vi "List Things.vi"(8 "error in (no error)":errorcluster, 11 "IoT Session in":refnum<class "IoT Session.lvclass">) -> (0 "error out":errorcluster, 2 "Things":string[](array[string]), 3 "IoT Session out":refnum<class "IoT Session.lvclass">)   [LabVIEW 2015, in "NI_AWS_IoT.lvlib" / "IoT Session.lvclass"]
uses:
  IoT Session.lvclass
  Core/HTTP Request/Request Options.ctl
  Core/HTTP Request/Name Value Pair.ctl
  Core/HTTP Request/Region handling.ctl
  Core/HTTP Request/URL formatting.ctl
  Core/HTTP Request/HTTP Request.lvclass
  JSON Parsing/NI_JSON Parsing.lvlib
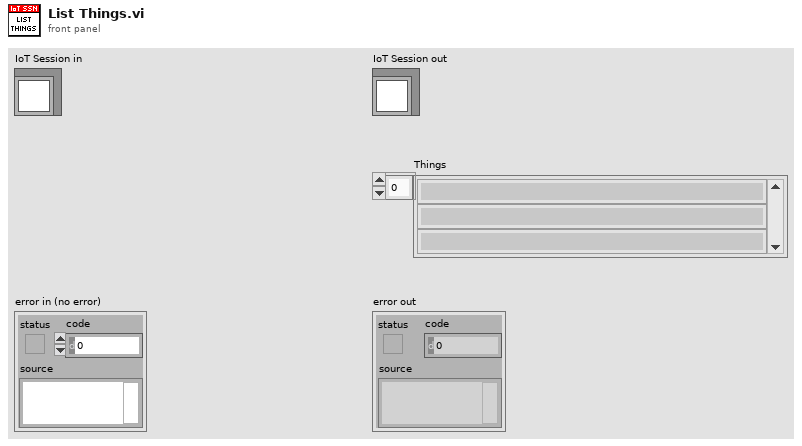
[diagram p1: front panel]
types:
  T1 = typedef "NI_AWS_Core.lvlib/HTTP Request.lvclass/Name Value Pair.ctl" = cluster{"name":string, "value":string}
  T2 = typedef "NI_AWS_Core.lvlib/HTTP Request.lvclass/Request Options.ctl" = cluster{"request headers":T1[], "request parameters":T1[], "request body":string, "region handling":T3, "URL formatting":T4}
  T3 = typedef "NI_AWS_Core.lvlib/HTTP Request.lvclass/Region handling.ctl" = enum16{"use region everywhere", "use region (authentication only)", "use region (URL only)", "ignore region everwhere"}
  T4 = typedef "NI_AWS_Core.lvlib/HTTP Request.lvclass/URL formatting.ctl" = enum16{"region-", "region."}
  T5 = typedef "NI_AWS_Core.lvlib/HTTP Request.lvclass/Response.ctl" = cluster{"Headers":string, "Body":string}
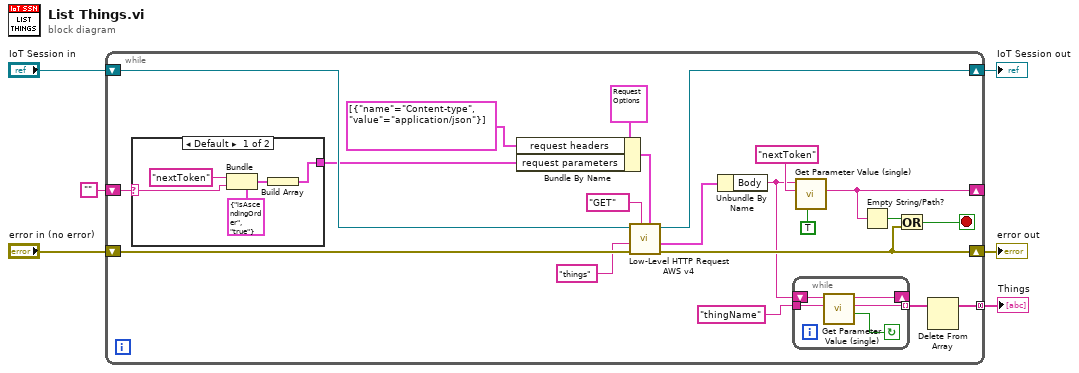
[diagram p0: block diagram]
diagram:
  n1 = while {
    shift-right: [w16] -> w5
    shift-left: "error in (no error)" -> [w24]
    shift-right: [w23] -> w4
    shift-left: "IoT Session in" -> [w22]
    shift-right: [w18] -> _
    shift-left: "" -> [w20]
    tunnel: [w7] -> w1 mode=concatenating
    stop <- w15 stop-if-true
    n2 = case shown="Default" w20 {
      selector: w20 -> [w34 _]
      tunnel: [w37 _] -> w12
      frame Default {
        n3 = Bundle(cluster=T1 {"name"="isAscendingOrder", "value"="true"} ("Name Value Pair"), "name"="nextToken", "value"=w34) -> (w35:T1)
        n4 = Build Array(w35) -> (w37:T1[])
      }
      frame "" {
      }
    }
    n5 = Bundle By Name(cluster=T2 {"request headers"=[], "request parameters"=[], "request body"="", "region handling"=enum."use region everywhere", "URL formatting"=enum."region."} ("Request Options"), "request headers"=T1[] [{"name"="Content-type", "value"="application/json"}], "request parameters"=w12) -> (w25:T2)
    n6 = call "Low-Level HTTP Request AWS v4.vi"("Request Options"=w25, "HTTP-Verb"="GET", "error in (no error)"=w24, "URL Suffix"="things" ("string"), "AWS Core in"=w22) -> ("error out"=w16:errorcluster, "Response"=w21:T5, "AWS Core out"=w23:refnum<class "IoT Session.lvclass">)  [unwired: 3 in, 1 out]
    n7 = Unbundle By Name(w21) -> ("Body"=w10:string)
    n8 = while {
      shift-right: [w30] -> _
      shift-left: w10 -> [w32]
      tunnel: "thingName" ("Parameter Name") -> [w31]
      tunnel: [w28] -> w8 mode=indexing
      stop <- w29 continue-if-true
      n9 = call "Get Parameter Value (single).vi"("Parameter Name"=w31, "JSON"=w32) -> ("Found"=w29:bool, "Parameter Value"=w28:string, "Remaining JSON"=w30:string)  [unwired: 6 in, 1 out]
    }
    n10 = call "Get Parameter Value (single).vi"("Clear Null"=TRUE, "Parameter Name"="nextToken", "JSON"=w10) -> ("Parameter Value"=w18:string)  [unwired: 5 in, 3 out]
    n11 = Empty String/Path?(string/path=w18) -> (empty?=w17:bool)
    n12 = Or(x=w17, y=w16) -> (x .or. y?=w15:bool)
    n13 = Delete From Array(array=w8) -> (array with subset deleted=w7:string[])  [unwired: 2 in, 1 out]
  }
  "error out" <- w5
  "IoT Session out" <- w4
  "Things" <- w1
